vi "New Person Object.vi"(7 "Person in":refnum<class "Person.lvclass">, 8 "error in (no error)":errorcluster, 9 "Date Of Birth":timestamp format="%<%x>T", 10 "Last Name":string, 11 "First Name":string) -> (0 "error out":errorcluster, 3 "Person out":refnum<class "Person.lvclass">)   [LabVIEW 2017, in "Person.lvclass"]
uses:
  Person.lvclass
  Person.lvclass/Person.ctl
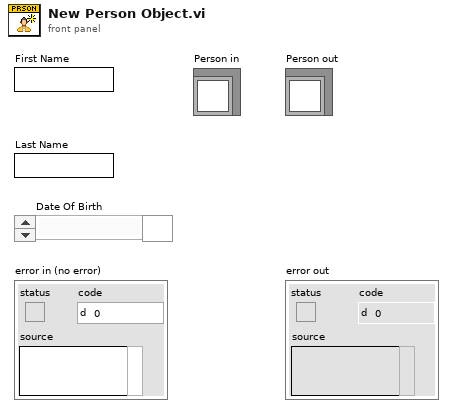
[diagram p1: front panel]
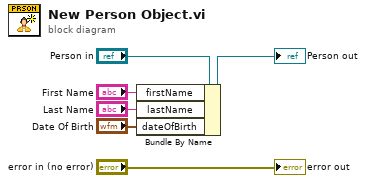
[diagram p0: block diagram]
diagram:
  n1 = Bundle By Name(cluster="Person in", "firstName"="First Name", "lastName"="Last Name", "dateOfBirth"="Date Of Birth") -> (→"Person out":refnum<class "Person.lvclass">)
  "error out" <- "error in (no error)"
